vi "Mcp2210 Set Spi Config.vi"(8 "error in (no error)":errorcluster, 10 "SPI Setting":T1 {"SPI Mode" items=["Mode 0", "Mode 1", "Mode 2", "Mode 3"]; "Baud Rate" format="%.0p"}, 11 "handle":i32) -> (0 "error out":errorcluster, 2 "SPI Setting Out":T1 {"SPI Mode" items=["Mode 0", "Mode 1", "Mode 2", "Mode 3"]; "Baud Rate" format="%.0p"}, 3 "handle out":i32)   [LabVIEW 2015, in "mcp2210.lvlib"]
doc: "Set the SPI transfer settings for current (VM) configuration or for power-up\ndefault (NVRAM) SPI configuration.\nIf SPI transfer is in progress, the configuration change is not accepted and the API returns\nE_ERR_SPI_CFG_ABORT error.\nIn the case of the current (VM) SPI configuration change, the API call returns the actual configuration\nvalues that will be used by the device, derived from the user supplied ones but adapted to the\ndevice capabilities.\nIf the NVRAM is password protected, the power-up SPI configuration cannot be changed and\nthe API returns E_ERR_BLOCKED_ACCESS error.\nParameters:\nInputs:\n- void *handle - The pointer to the device handle. Cannot be NULL.\n- unsigned char cfgSelector - current/power-up chip setting selection. Valid values are:\n- MCP2210_VM_CONFIG: designates current chip setting (Volatile\nMemory)\n- MCP2210_NVRAM_CONFIG: designates power-up chip setting (NVRAM)\nInputs / Outputs:\n- unsigned int *pbaudRate - transfer speed. Cannot be NULL.\n- unsigned int *pidleCsVal - IDLE chip select value. Cannot be NULL.\nbit31 - - - - bit8 bit0\nx x ... x x CS8 CS7 CS6 CS5 CS4 CS3 CS2 CS1 CS0\n- unsigned int *pactiveCsVal - Active Chip Select Value. Cannot be NULL.\nbit31 - - - - bit8 bit0\nx x ... x x CS8 CS7 CS6 CS5 CS4 CS3 CS2 CS1 CS0\n- unsigned int *pCsToDataDly - Chip Select to Data Delay (quanta of 100 us)\n- 16-bit value => max value is (2^16-1).\n- Cannot be NULL.\n- unsigned int *pdataToCsDly - Last Data Byte to CS (de-asserted) Delay (quanta of 100 us)\n- 16-bit value => max value is (2^16)-1.\n- Cannot be NULL.\n- unsigned int *pdataToDataDly - Delay Between Subsequent Data Bytes (quanta of 100 us)\n- 16-bit value => max value is (2^16)-1.\n- Cannot be NULL.\n- unsigned int *ptxferSize - Bytes to Transfer per SPI Transaction.\n- 16-bit value => max value is (2^16)-1.\n- Cannot be NULL.\n- unsigned char *pspiMd - SPI Mode. Cannot be NULL.\nValid values are:\n- MCP2210_SPI_MODE0\n- MCP2210_SPI_MODE1\n- MCP2210_SPI_MODE2\n- MCP2210_SPI_MODE3\nReturns:\n- 0 for success: E_SUCCESS\n- negative error code: E_ERR_NULL, E_ERR_INVALID_HANDLE_VALUE\nE_ERR_UNKOWN_ERROR, E_ERR_INVALID_PARAMETER\nE_ERR_HID_TIMEOUT, E_ERR_HID_RW_FILEIO\nE_ERR_BLOCKED_ACCESS, E_ERR_SPI_CFG_ABORT\n\nMCP2210_DLL_UM_API int __stdcall Mcp2210_SetSpiConfig(void *handle, unsigned char cfgSelector, unsigned int *pbaudRate, unsigned int *pidleCsVal,\n unsigned int *pactiveCsVal, unsigned int *pCsToDataDly, unsigned int *pdataToCsDly,\n unsigned int *pdataToDataDly, unsigned int *ptxferSize, unsigned char *pspiMd);"
uses:
  <userlib>/mcp2210/mcp2210.lvlib
  <userlib>/mcp2210/mcp2210_dll_um_x86.dll
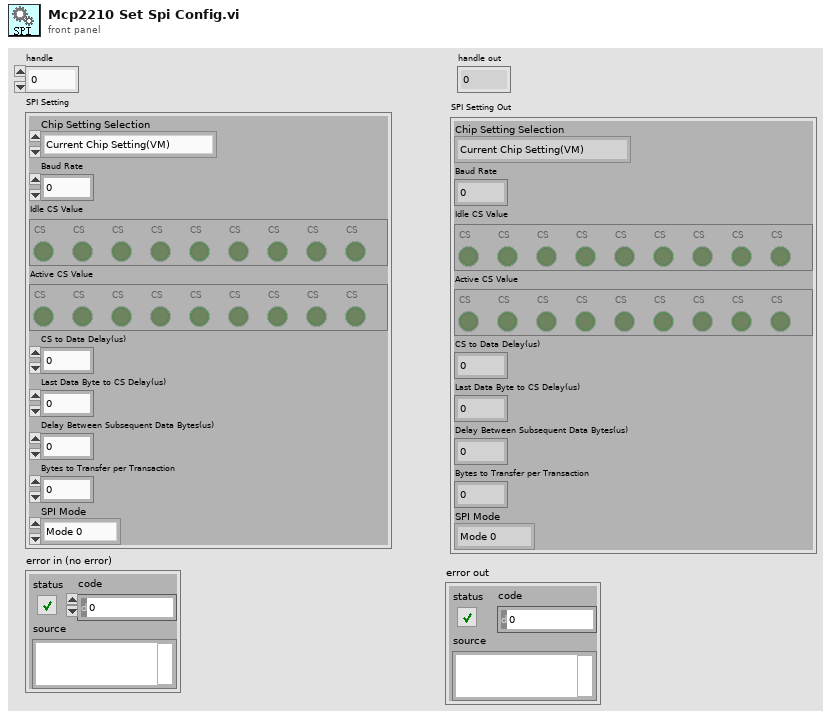
[diagram p1: front panel]
types:
  T1 = cluster{"Chip Setting Selection":enum8{"Current Chip Setting(VM)", "Power-up Chip Setting(NVRAM)"}, "Baud Rate":u32, "Idle CS Value":bool[], "Active CS Value":bool[], "CS to Data Delay(us)":u32, "Last Data Byte to CS Delay(us)":u32, "Delay Between Subsequent Data Bytes(us)":u32, "Bytes to Transfer per Transaction":u32, "SPI Mode":u8}
  T2 = enum8{"Current Chip Setting(VM)", "Power-up Chip Setting(NVRAM)"}
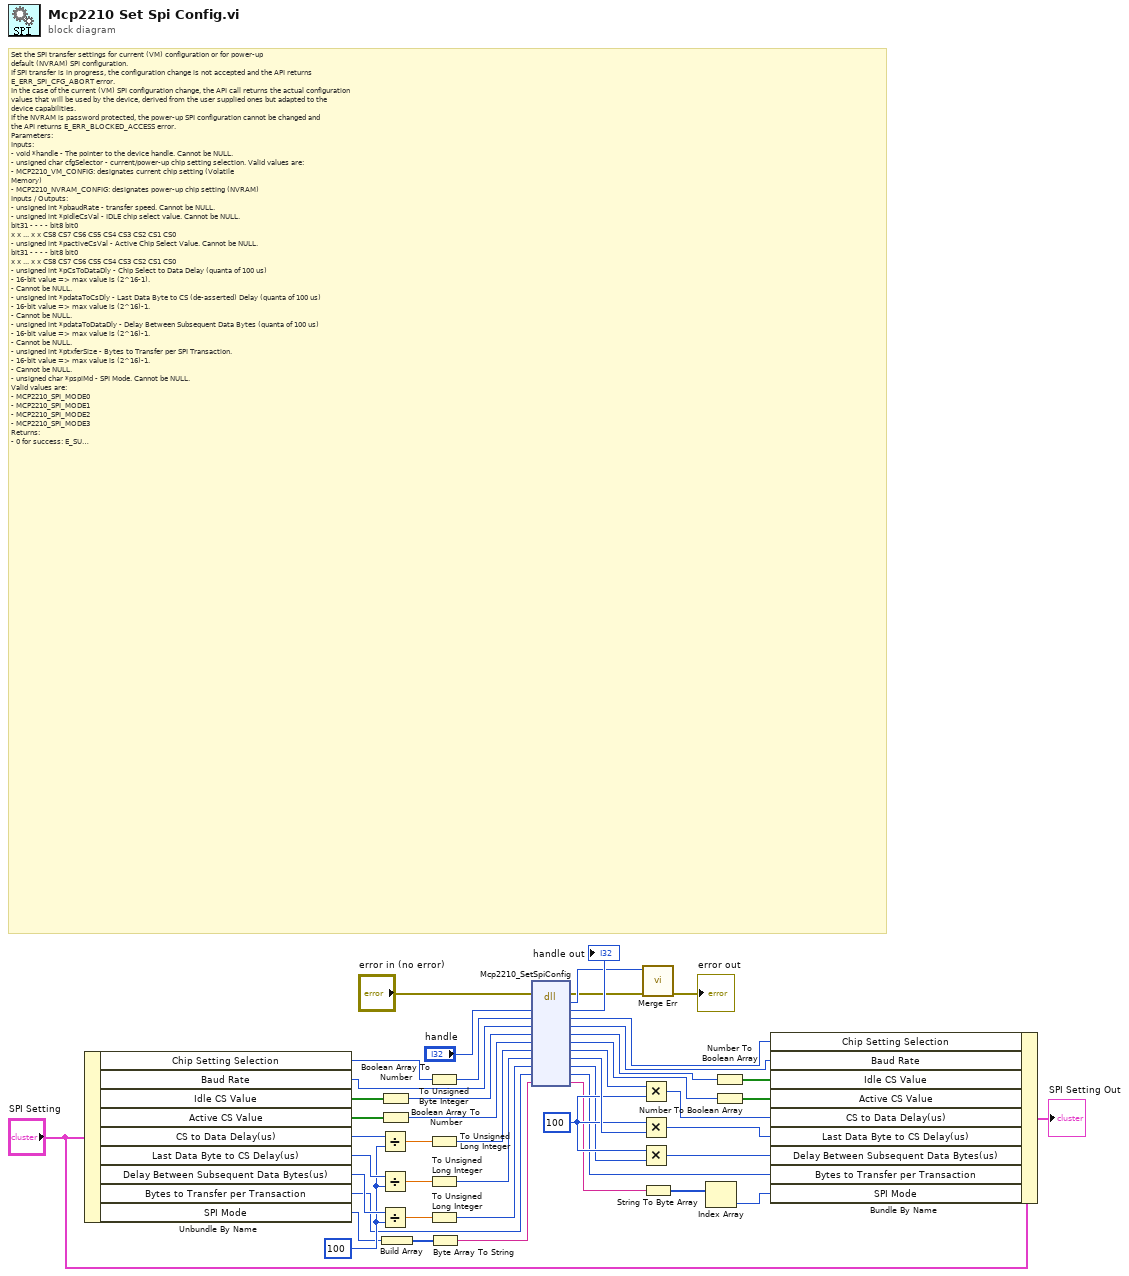
[diagram p0: block diagram]
diagram:
  w12 = u32 100 ("y")
  w31 = u32 100 ("y")
  # "Set the SPI transfer settings for current (VM) configuration or for power-up\ndefault (NVRAM) SPI configuration.\nIf SPI transfer is in progress, the configuration change is not accepted and the API returns\nE_ERR_SPI_CFG_ABORT error.\nIn the case of the current (VM) SPI configuration change, the API call returns the actual configuration\nvalues that will be used by the device, derived from the user supplied ones but adapted to the\ndevice capabilities.\nIf the NVRAM is password protected, the power-up SPI configuration cannot be changed and\nthe API returns E_ERR_BLOCKED_ACCESS error.\nParameters:\nInputs:\n- void *handle - The pointer to the device handle. Cannot be NULL.\n- unsigned char cfgSelector - current/power-up chip setting selection. Valid values are:\n- MCP2210_VM_CONFIG: designates current chip setting (Volatile\nMemory)\n- MCP2210_NVRAM_CONFIG: designates power-up chip setting (NVRAM)\nInputs / Outputs:\n- unsigned int *pbaudRate - transfer speed. Cannot be NULL.\n- unsigned int *pidleCsVal - IDLE chip select value. Cannot be NULL.\nbit31 - - - - bit8 bit0\nx x ... x x CS8 CS7 CS6 CS5 CS4 CS3 CS2 CS1 CS0\n- unsigned int *pactiveCsVal - Active Chip Select Value. Cannot be NULL.\nbit31 - - - - bit8 bit0\nx x ... x x CS8 CS7 CS6 CS5 CS4 CS3 CS2 CS1 CS0\n- unsigned int *pCsToDataDly - Chip Select to Data Delay (quanta of 100 us)\n- 16-bit value => max value is (2^16-1).\n- Cannot be NULL.\n- unsigned int *pdataToCsDly - Last Data Byte to CS (de-asserted) Delay (quanta of 100 us)\n- 16-bit value => max value is (2^16)-1.\n- Cannot be NULL.\n- unsigned int *pdataToDataDly - Delay Between Subsequent Data Bytes (quanta of 100 us)\n- 16-bit value => max value is (2^16)-1.\n- Cannot be NULL.\n- unsigned int *ptxferSize - Bytes to Transfer per SPI Transaction.\n- 16-bit value => max value is (2^16)-1.\n- Cannot be NULL.\n- unsigned char *pspiMd - SPI Mode. Cannot be NULL.\nValid values are:\n- MCP2210_SPI_MODE0\n- MCP2210_SPI_MODE1\n- MCP2210_SPI_MODE2\n- MCP2210_SPI_MODE3\nReturns:\n- 0 for success: E_SUCCESS\n- negative error code: E_ERR_NULL, E_ERR_INVALID_HANDLE_VALUE\nE_ERR_UNKOWN_ERROR, E_ERR_INVALID_PARAMETER\nE_ERR_HID_TIMEOUT, E_ERR_HID_RW_FILEIO\nE_ERR_BLOCKED_ACCESS, E_ERR_SPI_CFG_ABORT\n\nMCP2210_DLL_UM_API int __stdcall Mcp2210_SetSpiConfig(void *handle, unsigned char cfgSelector, unsigned int *pbaudRate, unsigned int *pidleCsVal,\n                                                      unsigned int *pactiveCsVal, unsigned int *pCsToDataDly, unsigned int *pdataToCsDly,\n                                                      unsigned int *pdataToDataDly, unsigned int *ptxferSize, unsigned char *pspiMd);"
  n1 = Unbundle By Name("SPI Setting") -> ("Chip Setting Selection"=w44:T2, "Baud Rate"=w43:u32, "Idle CS Value"=w42:bool[], "Active CS Value"=w40:bool[], "CS to Data Delay(us)"=w38:u32, "Last Data Byte to CS Delay(us)"=w35:u32, "Delay Between Subsequent Data Bytes(us)"=w32:u32, "Bytes to Transfer per Transaction"=w28:u32, "SPI Mode"=w27:u8)
  n2 = Divide(x=w38, y=w31) -> (x/y=w37:dbl)
  n3 = Divide(x=w35, y=w31) -> (x/y=w34:dbl)
  n4 = Divide(x=w32, y=w31) -> (x/y=w30:dbl)
  n5 = Boolean Array To Number(Boolean array=w42) -> (number=w41:u32)
  n6 = Boolean Array To Number(Boolean array=w40) -> (number=w39:u32)
  n7 = Build Array(w27) -> (w26:u8[])
  n8 = To Unsigned Byte Integer(number=w44) -> (unsigned 8bit integer=w23:u8)
  n9 = To Unsigned Long Integer(number=w37) -> (unsigned 32bit integer=w36:u32)
  n10 = To Unsigned Long Integer(number=w34) -> (unsigned 32bit integer=w33:u32)
  n11 = To Unsigned Long Integer(number=w30) -> (unsigned 32bit integer=w29:u32)
  n12 = Byte Array To String(unsigned byte array=w26) -> (string=w25:string)
  n13 = dll-call lib="D:/LabVIEW 2015/user.lib/mcp2210/mcp2210_dll_um_x86.*" fn="Mcp2210_SetSpiConfig"(error in="error in (no error)", "handle"="handle", "cfgSelector"=w23, "pbaudRate"=w43, "pidleCsVal"=w41, "pactiveCsVal"=w39, "pCsToDataDly"=w36, "pdataToCsDly"=w33, "pdataToDataDly"=w29, "ptxferSize"=w28, "pspiMd"=w25) -> (error out=w3:errorcluster, "return type"=w4:i32, "handle"=→"handle out":i32, "cfgSelector"=w22:u8, "pbaudRate"=w21:u32, "pidleCsVal"=w20:u32, "pactiveCsVal"=w17:u32, "pCsToDataDly"=w16:u32, "pdataToCsDly"=w13:u32, "pdataToDataDly"=w11:u32, "ptxferSize"=w10:u32, "pspiMd"=w8:string)  [unwired: 2 in, 1 out]
  n14 = Multiply(x=w16, y=w12) -> (x*y=w15:u32)
  n15 = Multiply(x=w12, y=w13) -> (x*y=w14:u32)
  n16 = Multiply(x=w12, y=w11) -> (x*y=w9:u32)
  n17 = call <userlib>:"Merge Err.vi"("error in (no error)"=w3, "return type"=w4) -> ("error out"=→"error out":errorcluster)  [unwired: 9 in]
  n18 = String To Byte Array(string=w8) -> (unsigned byte array=w7:u8[])
  n19 = Index Array(array=w7) -> (element=w6:u8)  [unwired: 1 in]
  n20 = Number To Boolean Array(number=w20) -> (Boolean array=w19:bool[])
  n21 = Number To Boolean Array(number=w17) -> (Boolean array=w18:bool[])
  n22 = Bundle By Name(cluster="SPI Setting", "Chip Setting Selection"=w22, "Baud Rate"=w21, "Idle CS Value"=w19, "Active CS Value"=w18, "CS to Data Delay(us)"=w15, "Last Data Byte to CS Delay(us)"=w14, "Delay Between Subsequent Data Bytes(us)"=w9, "Bytes to Transfer per Transaction"=w10, "SPI Mode"=w6) -> (→"SPI Setting Out":T1)
